vi "Create Error Queue.vi"(7 "max queue size (10)":u32=10, 8 "error in (no error)":errorcluster, 11 "error size":T1) -> (0 "error out":errorcluster, 3 "Error Queue":T2)   [LabVIEW 2017, in "Data Sharing Framework Core.lvlib" / "Data Sharing Framework Engine.lvlib" / "Engine Interface.lvclass"]
uses:
  Engine Interface.lvclass
  Error Queue Ref.ctl
  Error Queue Sizes.ctl
  <vilib>/NI/Memory Manager/VIs/New Error Cluster Constant (256B).vi
  <vilib>/NI/Memory Manager/VIs/New Error Cluster Constant (512B).vi
  <vilib>/NI/Memory Manager/VIs/New Error Cluster Constant (1024B).vi
  <vilib>/NI/Memory Manager/VIs/Source.Write.String.vi
  <vilib>/NI/Memory Manager/Static Error Handling.lvlib
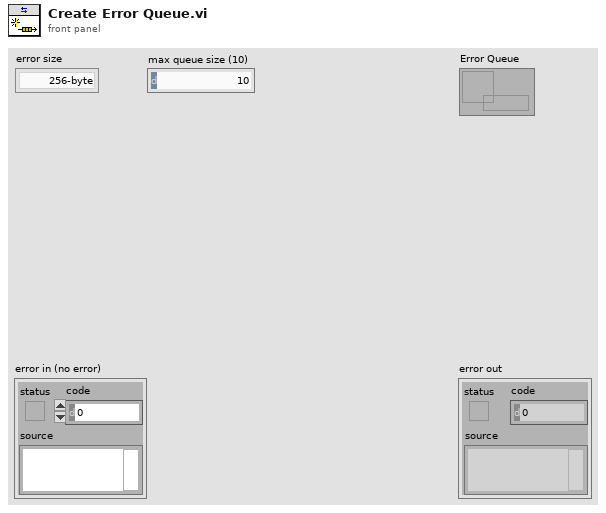
[diagram p1: front panel]
types:
  T1 = typedef "Data Sharing Framework Core.lvlib/Data Sharing Framework Engine.lvlib/Engine Interface.lvclass/Error Queue Sizes.ctl" = enum16{"256-byte", "512-byte", "1024-byte"}
  T2 = typedef "Data Sharing Framework Core.lvlib/Data Sharing Framework Engine.lvlib/Engine Interface.lvclass/Error Queue Ref.ctl" = refnum<queue>
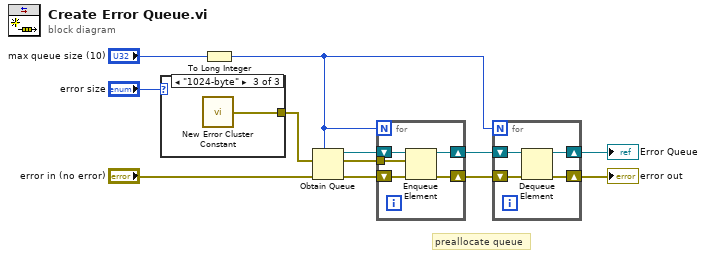
[diagram p0: block diagram]
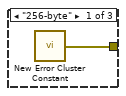
[diagram p2: hidden frame]
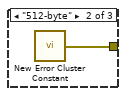
[diagram p3: hidden frame]
diagram:
  # "preallocate queue"
  n1 = case shown="\"1024-byte\"" "error size" {
    tunnel: [w12 w13 w14] -> w3
    frame "256-byte" {
      n2 = call-poly <vilib>:"New Error Cluster Constant.vi"() -> ("error out"=w12:errorcluster)  [unwired: 1 in]
    }
    frame "512-byte" {
      n3 = call-poly <vilib>:"New Error Cluster Constant.vi"() -> ("error out"=w13:errorcluster)  [unwired: 1 in]
    }
    frame "1024-byte" {
      n4 = call-poly <vilib>:"New Error Cluster Constant.vi"() -> ("error out"=w14:errorcluster)  [unwired: 1 in]
    }
  }
  n5 = To Long Integer(number="max queue size (10)") -> (32bit integer=w1:i32)
  n6 = Obtain Queue(max queue size (-1, unlimited)=w1, element data type=w3, error in (no error)="error in (no error)") -> (queue out=w9:refnum<queue>, error out=w8:errorcluster)  [unwired: 2 in, 1 out]
  n7 = for {
    N: w1 -> [_]
    shift-right: [w17] -> w7
    shift-left: w9 -> [w19]
    shift-right: [w16] -> w6
    shift-left: w8 -> [w18]
    tunnel: w3 -> [w15]
    n8 = Enqueue Element(queue=w19, element=w15, error in (no error)=w18) -> (queue out=w17:refnum<queue>, error out=w16:errorcluster)  [unwired: 1 in, 1 out]
  }
  n9 = for {
    N: w1 -> [_]
    shift-right: [w21] -> w5
    shift-left: w7 -> [w23]
    shift-right: [w20] -> w4
    shift-left: w6 -> [w22]
    n10 = Dequeue Element(queue=w23, error in (no error)=w22) -> (queue out=w21:refnum<queue>, error out=w20:errorcluster)  [unwired: 1 in, 2 out]
  }
  "error out" <- w4
  "Error Queue" <- w5
